vi "Report Startup to Process.vi"(8 "Error":errorcluster, 11 "This VI":refnum<vi>) -> (0 "error out":errorcluster)   [LabVIEW 2015, in "Control Addon Engine.lvlib" / "Error Handling API.lvlib"]
uses:
  Error Handling API.lvlib
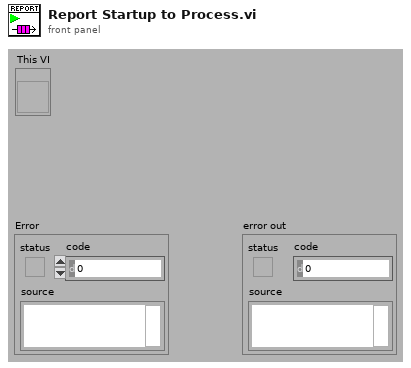
[diagram p1: front panel]
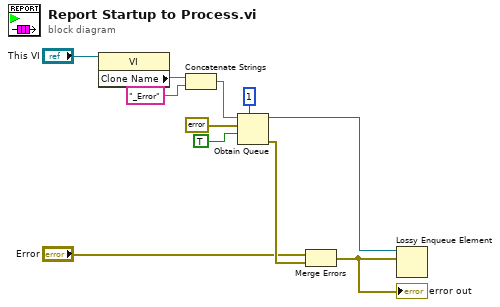
[diagram p0: block diagram]
diagram:
  n1 = property class="VI"(reference="This VI") -> ("Clone Name"=w9:string)  [unwired: 1 in, 2 out]
  n2 = Concatenate Strings(w9, "_Error" ("string")) -> (w7:string)
  n3 = Obtain Queue(max queue size (-1, unlimited)=1, name (unnamed)=w7, element data type=errorcluster {"status"=FALSE, "code"=0, "source"=""} ("error out"), create if not found? (T)=TRUE) -> (queue out=w10:refnum<queue>, error out=w3:errorcluster)  [unwired: 1 in, 1 out]
  n4 = Merge Errors("Error", w3) -> (w1:errorcluster)
  "error out" <- w1
  n5 = Lossy Enqueue Element(queue=w10, element=w1) -> ()  [unwired: 1 in, 4 out]
